vi "LinVer Daten verwalten.vi"(6 "Aktionen":T6, 7 "Dateiname":string, 8 "Pfad":string, 9 "Stufen Tabelle":T5, 11 "Lin Daten":T1 {"CalGas Eingang" items=["Cal Gas 1", "Cal Gas 2", "Cal Gas 3"]; "Max Fehler (Sollwert)" format="%#_5g"; "Zeitdauer Stufe" format="%#_5g"; "Anzahl Stufen" format="%#_5g"; "Verdünnungsgas" items=["N2", "O2"]}) -> (0 "Pfad":string, 1 "Stufen Tabelle":T5, 2 "Lin Daten einzeln":T1 {"CalGas Eingang" items=["Cal Gas 1", "Cal Gas 2", "Cal Gas 3"]; "Max Fehler (Sollwert)" format="%#_5g"; "Zeitdauer Stufe" format="%#_5g"; "Anzahl Stufen" format="%#_5g"; "Verdünnungsgas" items=["N2", "O2"]}, 3 "Gefunden?":bool, 5 "Dateiname":string)   [LabVIEW 2015, in "Linearisierung v2.lvlib" / "Linearity verification 1065-307.lvlib"]
uses:
  Linearity verification 1065-307.lvlib
  Visualisierungs Elemente/String - Eingabefeld.ctl
  Visualisierungs Elemente/Zahlen-Eingabefeld.ctl
  Gasteiler/Lin Daten.ctl
  Gasteiler/Gasteiler.lvlib
  Gasteiler/Stufen Tabelle.ctl
  LinVer Daten verwalten Aktionen.ctl
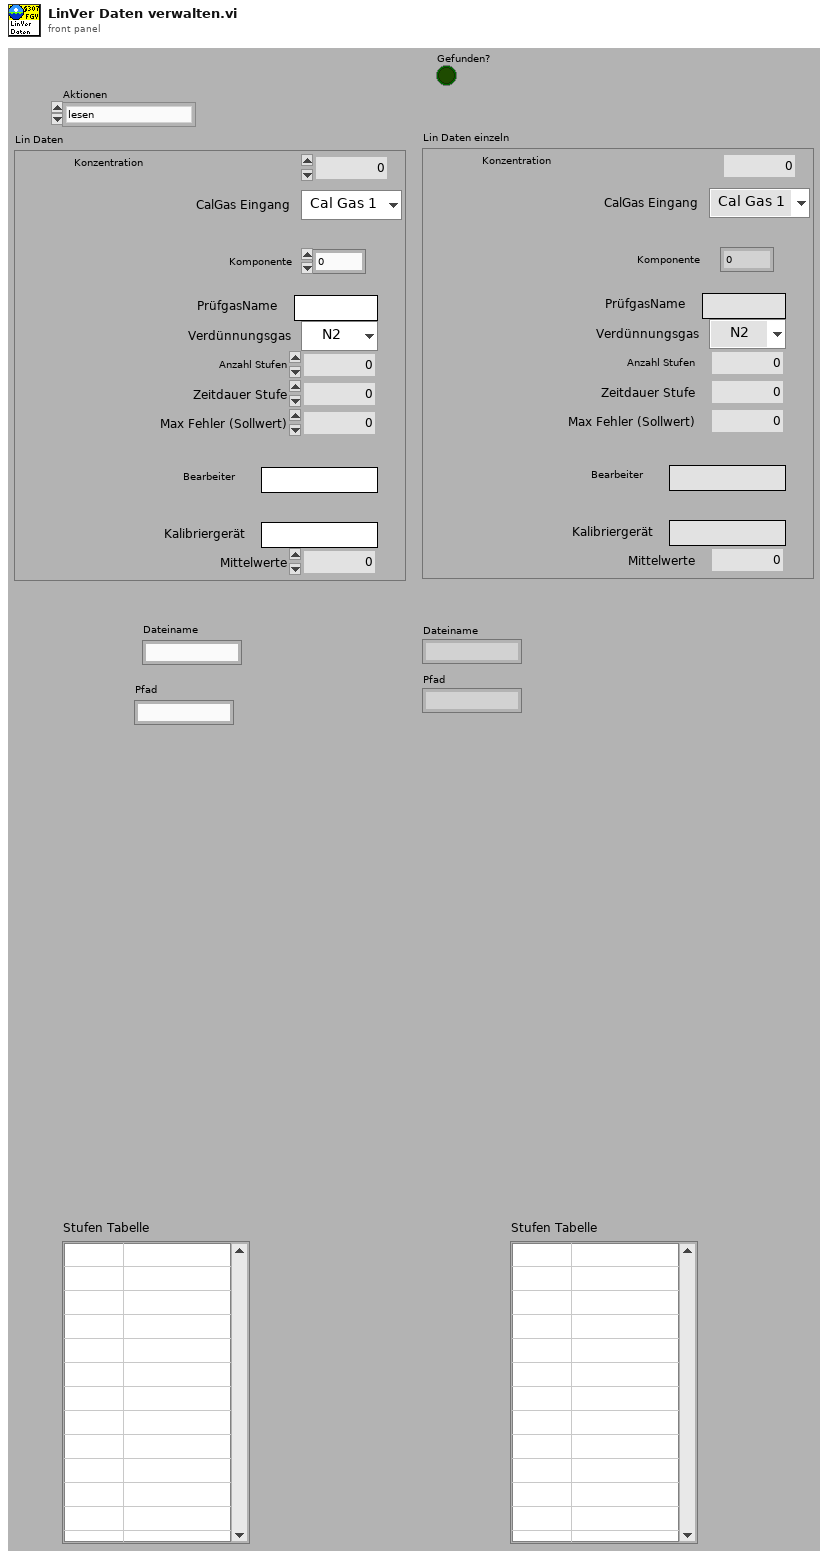
[diagram p1: front panel]
types:
  T1 = typedef "Linearisierung v2.lvlib/Gasteiler.lvlib/Lin Daten.ctl" = cluster{"PrüfgasName":T2, "Verdünnungsgas":T3, "Anzahl Stufen":T4, "Zeitdauer Stufe":T4, "Max Fehler (Sollwert)":T4, "Bearbeiter":T2, "Kalibriergerät":T2, "Mittelwerte":i32, "Komponente":u16, "CalGas Eingang":u16, "Konzentration":sgl}
  T2 = typedef "String - Eingabefeld.ctl" = string
  T3 = typedef "Linearisierung v2.lvlib/Gasteiler.lvlib/Prüfgas in.ctl" = u16
  T4 = typedef "Zahlen-Eingabefeld.ctl" = sgl
  T5 = typedef "Linearisierung v2.lvlib/Gasteiler.lvlib/Stufen Tabelle.ctl" = string[][]
  T6 = typedef "Linearisierung v2.lvlib/Linearity verification 1065-307.lvlib/LinVer Daten verwalten Aktionen.ctl" = enum16{"lesen", "speichern", "laden", "Lin Daten schr.", "Stufen Tabelle", "Lin Name AK", "Lin Pfad AK"}
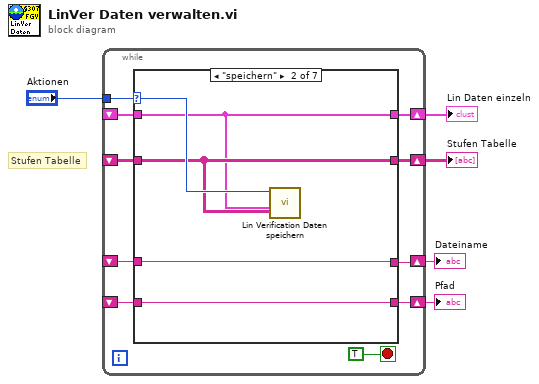
[diagram p0: block diagram]
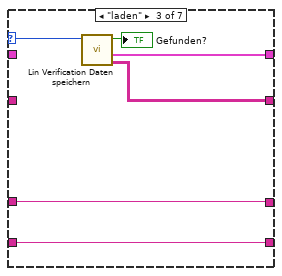
[diagram p3: hidden frame]
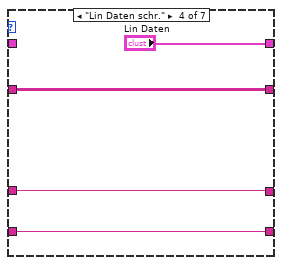
[diagram p4: hidden frame]
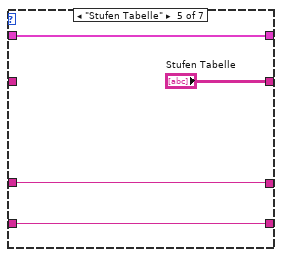
[diagram p5: hidden frame]
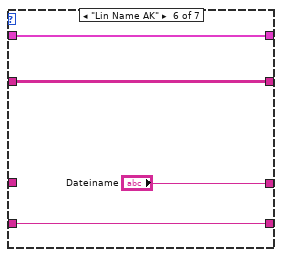
[diagram p6: hidden frame]
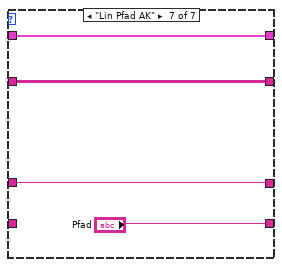
[diagram p7: hidden frame]
diagram:
  # "Stufen Tabelle"
  n1 = while {
    tunnel: "Aktionen" -> [w14]
    shift-right: [w13] -> w4
    shift-left: _ -> [w12]
    shift-right: [w10] -> w3
    shift-left: _ -> [w11]
    shift-right: [w9] -> w2
    shift-left: _ -> [w8]
    shift-right: [w7] -> w1
    shift-left: _ -> [w6]
    stop <- TRUE stop-if-true
    n2 = case shown="\"speichern\"" w14 {
      selector: w14 -> [_ w24 w30 _ _ _ _]
      tunnel: [w19 w22 w28 "Lin Daten" w38 w42 w44] -> w13
      tunnel: w12 -> [w19 w22 _ _ w38 w42 w44]
      tunnel: w11 -> [w18 w23 _ w34 _ w41 w45]
      tunnel: [w18 w23 w29 w34 "Stufen Tabelle" w41 w45] -> w10
      tunnel: [w17 w21 w27 w32 w36 "Dateiname" w46] -> w9
      tunnel: w8 -> [w17 w21 w27 w32 w36 _ w46]
      tunnel: [w16 w20 w26 w31 w35 w39 "Pfad"] -> w7
      tunnel: w6 -> [w16 w20 w26 w31 w35 w39 _]
      frame "lesen", Default {
      }
      frame "speichern" {
        n3 = call "Lin Verification Daten speichern.vi"("Stufen Tabelle"=w23, "Lin Daten"=w22, "Aktionen"=w24) -> ()  [unwired: 6 in, 3 out]
      }
      frame "laden" {
        n4 = call "Lin Verification Daten speichern.vi"("Aktionen"=w30) -> ("Stufen Tabellen"=w29:T5, "Lin Daten Array"=w28:T1, "Gefunden?"=→"Gefunden?":bool)  [unwired: 8 in]
      }
      frame "Lin Daten schr." {
      }
      frame "Stufen Tabelle" {
      }
      frame "Lin Name AK" {
      }
      frame "Lin Pfad AK" {
      }
    }
  }
  "Lin Daten einzeln" <- w4
  "Stufen Tabelle" <- w3
  "Dateiname" <- w2
  "Pfad" <- w1
